vi "MultiplexerSerialInterface.vi"() -> ()   [LabVIEW 2016]
uses:
  <vilib>/rvi/interface/nirviOpenFPGA/nirviOpenFPGA.xnode
  <vilib>/rvi/interface/nirviReadWriteControl/nirviReadWriteControl.xnode
  FPGA Bitfiles/qnmController797_usbRIO_MultiplexerSeria_ssMkrCMtubE.lvbitx
  <vilib>/FPGAPlugInAG/USB-7856R OEM/niLvFpga_Open_USB-7856R OEM.vi
  <vilib>/rvi/interface/common/dynamic/niFpgaDynamicAddResources.vi
  <vilib>/rvi/interface/Simulation/niFpgaSimulationCallBeginRW.vi
  <vilib>/rvi/errors/niLvFpgaAdjustHostInterfaceError.vi
panel:
  in  "Sequence number":i32
  in  "Delay between pts":u32=10000
  in  "Update (ms)":u32
  in  "stop":bool
  out "Waveform Chart":i16(graph)
  in  "Sequence":bool[][](array[boolean])
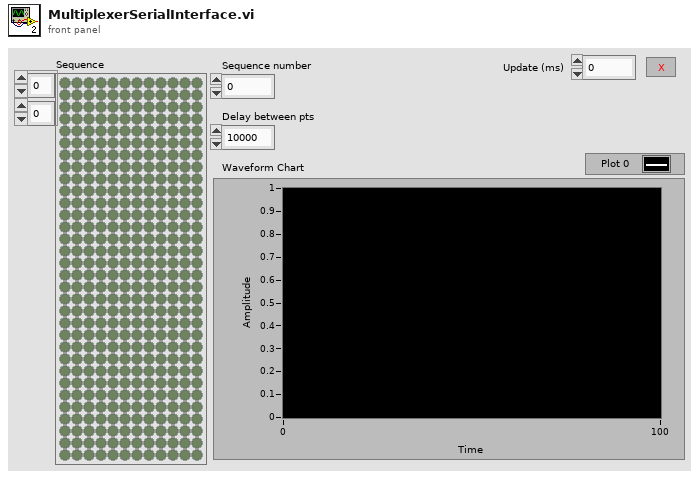
[diagram p1: front panel]
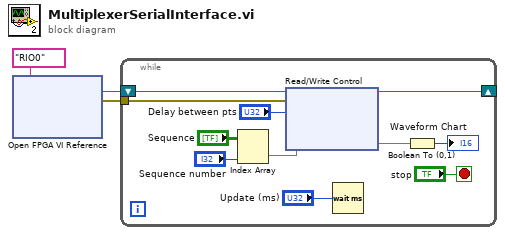
[diagram p0: block diagram]
diagram:
  n1 = xnode "Open FPGA VI Reference"("resource name"=tag "RIO0") -> ("FPGA VI Reference Out"=w2:refnum<k20>, "error out"=w3:errorcluster)  [unwired: 1 in]
  n2 = while {
    tunnel: w3 -> [w13]
    shift-right: [w12] -> _
    shift-left: w2 -> [w14]
    stop <- "stop" stop-if-true
    n3 = Index Array(array="Sequence", index (col)="Sequence number") -> (element=w5:bool[])  [unwired: 1 in]
    n4 = xnode "Read/Write Control"("FPGA VI Reference In"=w14, "error in"=w13, "Count(mSec)"="Delay between pts", "Data In (DIO8)"=w5) -> ("FPGA VI Reference Out"=w12:refnum<k20>, "DIO8"=w4)  [unwired: 1 out]
    n5 = Wait (ms)(milliseconds to wait="Update (ms)") -> ()  [unwired: 1 out]
    n6 = Boolean To (0,1)(Boolean=w4) -> (0, 1=→"Waveform Chart":i16)
  }
